vi "GetType.vi"(8 "error in (no error)":errorcluster, 11 "Selftest Device Msg in":refnum<class "Selftest Device Msg.lvclass">) -> (0 "error out":errorcluster, 2 "Data Sample":variant, 3 "Selftest Device Msg out":refnum<class "Selftest Device Msg.lvclass">)   [LabVIEW 2014, in "CS++DeviceActor.lvlib" / "Selftest Device Msg.lvclass"]
doc: "This VI delivers a sample of the data type format the message expects."
uses:
  Selftest Device Msg.lvclass
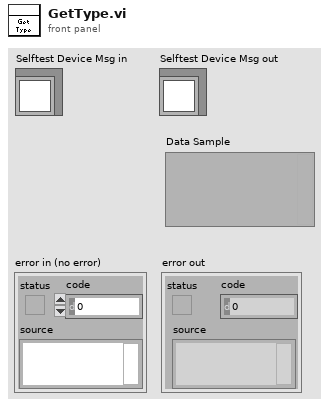
[diagram p1: front panel]
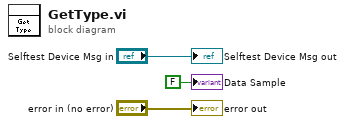
[diagram p0: block diagram]
diagram:
  "error out" <- "error in (no error)"
  "Selftest Device Msg out" <- "Selftest Device Msg in"
  "Data Sample" <- FALSE
